vi "ReadConfig.vi"(0 "reference in":refnum<class "NodeConfiguration.lvclass">, 5 "error in (no error)":errorcluster) -> (14 "reference out":refnum<class "NodeConfiguration.lvclass">, 16 "Config":T1, 19 "error out":errorcluster)   [LabVIEW 2014, in "NodeConfiguration.lvclass"]
uses:
  NodeConfiguration.lvclass
  Config.ctl
  <vilib>/Utility/config.llb/NI_LVConfig.lvlib
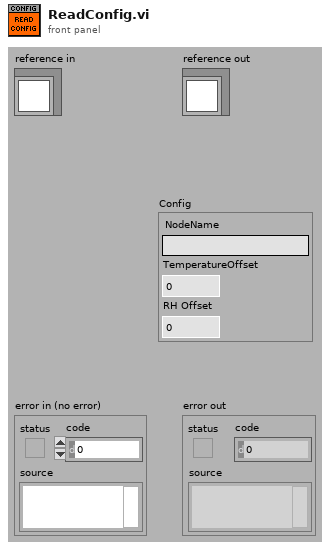
[diagram p1: front panel]
types:
  T1 = typedef "NodeConfiguration.lvclass/Config.ctl" = cluster{"NodeName":string, "TemperatureOffset":dbl, "RH Offset":dbl}
  T2 = typedef "NodeConfiguration.lvclass/ObjectAttributes.ctl" = cluster{"Config":T1, "ConfigFile":path}
  T3 = typedef "NI_LVConfig.lvlib/Config Data RefNum.ctl" = refnum<k1>
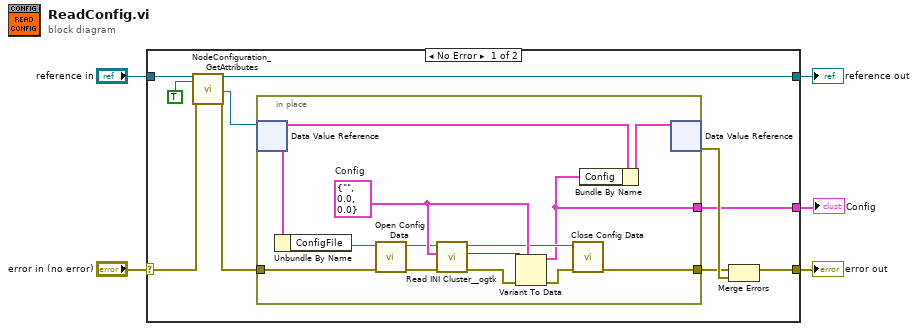
[diagram p0: block diagram]
diagram:
  n1 = case shown="No Error" "error in (no error)" {
    selector: "error in (no error)" -> [w12 w30]
    tunnel: [w14 w30] -> w4
    tunnel: [w10 w29] -> w2
    tunnel: "reference in" -> [w13 w29]
    tunnel: [w6 _] -> w1
    frame No Error {
      n2 = call "NodeConfiguration_GetAttributes.vi"("reference in"=w13, "OnlyGetDvrReference(False)"=TRUE, "error in (no error)"=w12) -> ("reference out"=w10:refnum<class "NodeConfiguration.lvclass">, "DataRef"=w11:refnum<data-value>, "error out"=w8:errorcluster)  [unwired: 13 in, 1 out]
      n3 = in-place {
        in-place-border: w8 -> [w26]
        in-place-border: [w24] -> w7
        in-place-border: [w16] -> w6
        w20 = T1 {"NodeName"="", "TemperatureOffset"=0.0, "RH Offset"=0.0}  # Config
        n4 = in-place-dvr #1(w11) -> (w27:T2)  [unwired: 1 out]
        n5 = Unbundle By Name(w27) -> ("ConfigFile"=w25:path)
        n6 = call <vilib>:"Open Config Data.vi"("error in (no error)"=w26, "configuration file path"=w25) -> ("error out"=w22:errorcluster, "refnum"=w19:T3)  [unwired: 7 in, 1 out]
        n7 = call <userlib>:"Read INI Cluster__ogtk.vi"("error in (no error)"=w22, "INI Fomatted Cluster Type"=w20, "refnum"=w19) -> ("error out"=w21:errorcluster, "INI Fomatted Cluster"=w17:variant, "dup refnum"=w18:T3)  [unwired: 4 in, 2 out]
        n8 = Variant To Data(error in=w21, type=w20, Variant=w17) -> (data=w16:T1, error out=w23:errorcluster)
        n9 = call <vilib>:"Close Config Data.vi"("error in (no error)"=w23, "refnum"=w18) -> ("error out"=w24:errorcluster)  [unwired: 8 in, 1 out]
        n10 = Bundle By Name(cluster=w27, "Config"=w16) -> (w28:T2)
        n11 = in-place-dvr #1(w28) -> (w15:errorcluster)  [unwired: 1 out]
      }
      n12 = Merge Errors(w7, w15) -> (w14:errorcluster)
    }
    frame Error {
    }
  }
  "error out" <- w4
  "reference out" <- w2
  "Config" <- w1
